vi "Formular Analyze.vi"(8 "error in (no error)":errorcluster caption="Error In", 10 "Formular":string="EL_A/(SY_Pieces*SY_Activation_Area)", 11 "Project":string) -> (0 "error out":errorcluster caption="Error Out", 1 "Value":string[](array[string]), 2 "Parameter":string[](array[string]), 3 "Result":string, 5 "Value":dbl)   [LabVIEW 2020]
uses:
  Global/Data Global/Data Global Mode.ctl
  375d7d93-2e26-4f59-bd85-31ccd4dbf3b0.vi
  <vilib>/regexp/Match Regular Expression.xnode
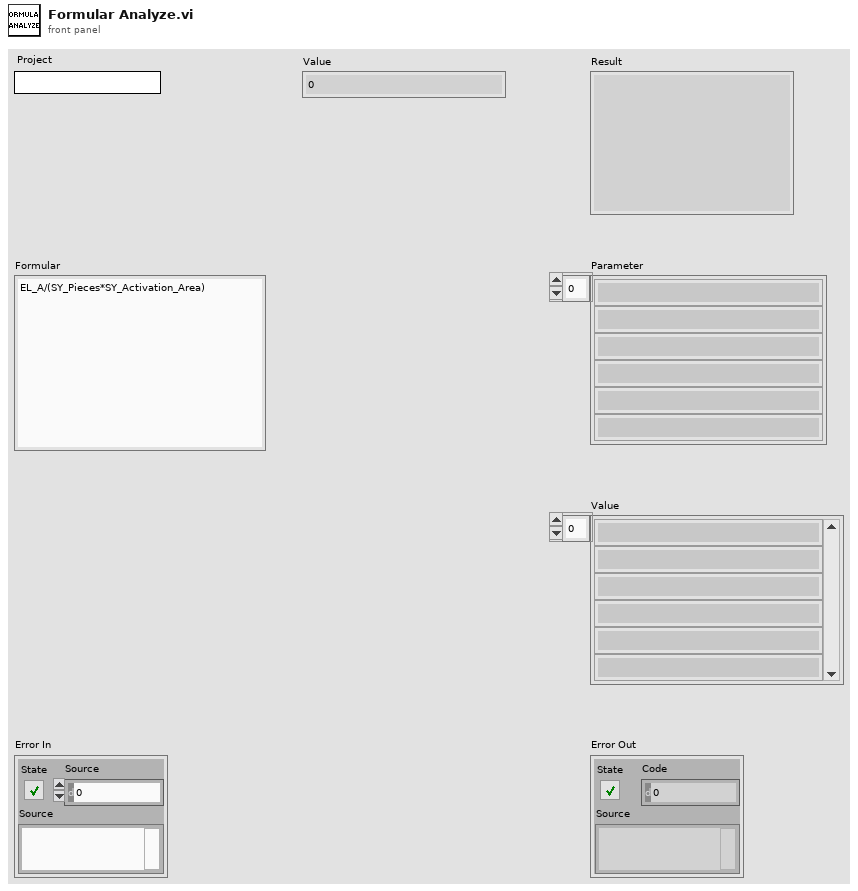
[diagram p1: front panel]
types:
  T1 = typedef "Data Global Mode.ctl" = enum16{"Init", "Read", "Write", "Write Data", "Load"}
  T2 = typedef "SDQ Data Type.ctl" = cluster{"CAN Length":string, "CAN Name":string, "CAN ID":string, "CAN Type":string, "Test Item":string, "Byte Order":string, "Instruction":string, "Control Type":string, "Group":string, "Offset":dbl, "Coefficient":dbl, "Write Enable":bool, "Lable Type":string, "Key?":string, "Set Value":string, "Upper":dbl, "Lower":dbl, "Unit":string, "Formula":string, "Test Item Type":string, "Length":i32, "Address":string, "Name":string, "Identifier":string, "Data Type":string, "Enumerate?":string, "Enumerate List":string, "Data":string, "Source":string}
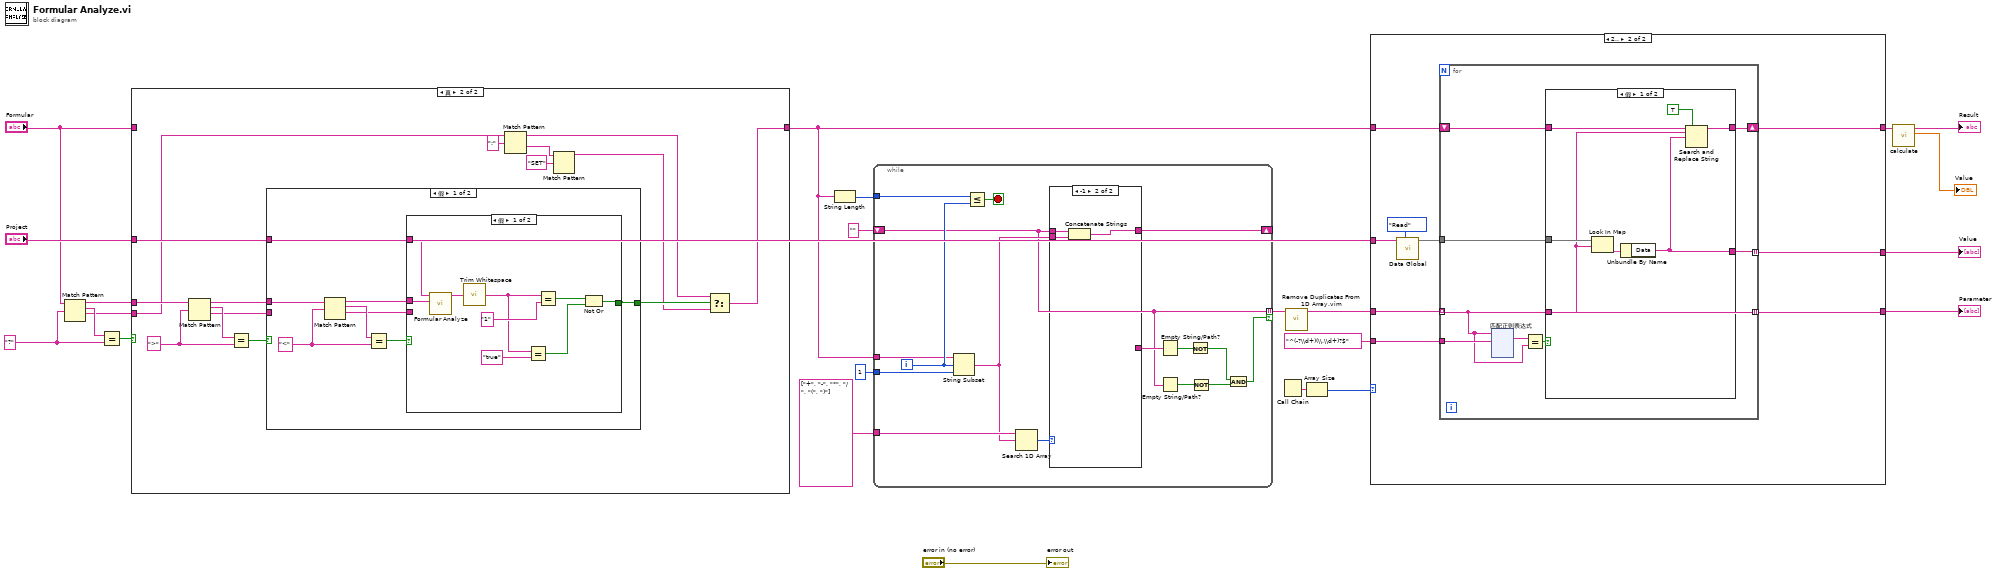
[diagram p0: block diagram]
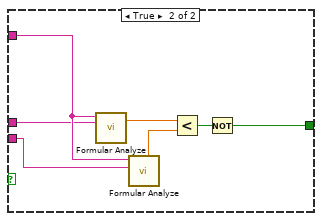
[diagram p3: hidden frame]
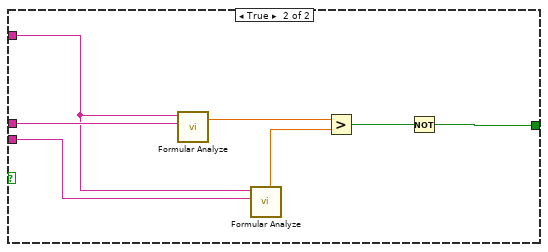
[diagram p4: hidden frame]
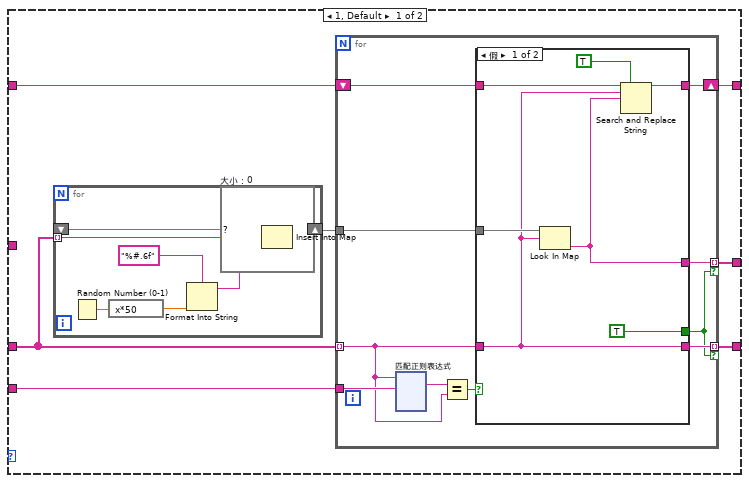
[diagram p5: hidden frame]
diagram:
  w10 = "?" ("正则表达式")
  n1 = Match Pattern(string="Formular", regular expression=w10) -> (before substring=w7:string, match substring=w11:string, after substring=w4:string)  [unwired: 1 in, 1 out]
  n2 = Equal?(x=w11, y=w10) -> (x = y?=w9:bool)
  n3 = case shown="真" w9 {
    tunnel: w7 -> [_ w39]
    tunnel: "Project" -> [_ w33]
    tunnel: w4 -> [_ w31]
    tunnel: "Formular" -> [w24 _]
    tunnel: [w24 w29] -> w2
    frame False {
    }
    frame True {
      w37 = ">" ("字符串")
      n4 = Match Pattern(string=w39, regular expression=w37) -> (before substring=w35:string, match substring=w38:string, after substring=w34:string)  [unwired: 1 in, 1 out]
      n5 = Equal?(x=w38, y=w37) -> (x = y?=w36:bool)
      n6 = case shown="假" w36 {
        tunnel: w35 -> [w47 w67]
        tunnel: w34 -> [_ w68]
        tunnel: w33 -> [w40 w66]
        tunnel: [w41 w64] -> w28
        frame False {
          w45 = "<" ("正则表达式")
          n7 = Match Pattern(string=w47, regular expression=w45) -> (before substring=w43:string, match substring=w46:string, after substring=w42:string)  [unwired: 1 in, 1 out]
          n8 = Equal?(x=w46, y=w45) -> (x = y?=w44:bool)
          n9 = case shown="假" w44 {
            tunnel: w43 -> [w49 w60]
            tunnel: w42 -> [_ w59]
            tunnel: [w52 w57] -> w41
            tunnel: w40 -> [w50 w61]
            frame False {
              n10 = call "Formular Analyze.vi"("Formular"=w49, "Project"=w50) -> ("Result"=w48:string)  [unwired: 5 in, 4 out]
              n11 = call <vilib>:"Trim Whitespace.vi"("string"=w48) -> ("trimmed string"=w51:string)  [unwired: 1 in]
              n12 = Equal?(x=w51, y="true") -> (x = y?=w53:bool)
              n13 = Equal?(x=w51, y="1") -> (x = y?=w54:bool)
              n14 = Not Or(1:w53, 2:w54) -> (0:w52:bool)
            }
            frame True {
              n15 = call "Formular Analyze.vi"("Formular"=w60, "Project"=w61) -> ("Value"=w63:dbl)  [unwired: 5 in, 4 out]
              n16 = call "Formular Analyze.vi"("Formular"=w59, "Project"=w61) -> ("Value"=w62:dbl)  [unwired: 5 in, 4 out]
              n17 = Less?(x=w63, y=w62) -> (x < y?=w58:bool)
              n18 = Not(x=w58) -> (.not. x?=w57:bool)
            }
          }
        }
        frame True {
          n19 = call "Formular Analyze.vi"("Formular"=w67, "Project"=w66) -> ("Value"=w70:dbl)  [unwired: 5 in, 4 out]
          n20 = call "Formular Analyze.vi"("Formular"=w68, "Project"=w66) -> ("Value"=w69:dbl)  [unwired: 5 in, 4 out]
          n21 = Greater?(x=w70, y=w69) -> (0:w65:bool)
          n22 = Not(x=w65) -> (.not. x?=w64:bool)
        }
      }
      n23 = Match Pattern(string=w31, regular expression=":" ("正则表达式")) -> (before substring=w30:string, after substring=w27:string)  [unwired: 1 in, 2 out]
      n24 = Match Pattern(string=w27, regular expression="SET" ("正则表达式")) -> (before substring=w25:string)  [unwired: 1 in, 3 out]
      n25 = Select(t=w30, s=w28, f=w25) -> (s? t:f=w29:string)
    }
  }
  n26 = String Length(string=w2) -> (length=w22:i32)
  n27 = while {
    tunnel: string[] ["+", "-", "*", "/", "(", ")"] -> [w82]
    tunnel: w22 -> [w86]
    tunnel: 1 ("长度（剩余）") -> [w83]
    shift-right: [w81] -> _
    shift-left: "" -> [w74]
    tunnel: [w74] -> w8 mode=indexing if=w72
    tunnel: w2 -> [w79]
    i -> [w84]
    stop <- w85 stop-if-true
    n28 = String Subset(string=w79, offset (0)=w84, length (rest)=w83) -> (substring=w77:string)
    n29 = Less Or Equal?(x=w86, y=w84) -> (x <= y?=w85:bool)
    n30 = Search 1D Array(1D array=w82, element=w77) -> (index of element=w78:i32)  [unwired: 1 in]
    n31 = case shown="-1" w78 {
      tunnel: w74 -> [_ w90]
      tunnel: w77 -> [w87 w89]
      tunnel: [_ w88] -> w81
      tunnel: [w87 _] -> w76
      frame 0, Default {
      }
      frame -1 {
        n32 = Concatenate Strings(w90, w89) -> (w88:string)
      }
    }
    n33 = Empty String/Path?(string/path=w76) -> (empty?=w80:bool)
    n34 = Empty String/Path?(string/path=w74) -> (empty?=w75:bool)
    n35 = Not(x=w80) -> (.not. x?=w71:bool)
    n36 = Not(x=w75) -> (.not. x?=w73:bool)
    n37 = And(x=w71, y=w73) -> (x .and. y?=w72:bool)
  }
  n38 = Call Chain() -> (call chain=w18:string[])
  n39 = call "Remove Duplicates From 1D Array.vim"("array"=w8) -> ("array with duplicates removed"=w15:string[])  [unwired: 10 in]
  n40 = Array Size(array=w18) -> (size(s)=w17:i32)
  n41 = case shown="2.." w17 {
    tunnel: w15 -> [w94 w245]
    tunnel: w2 -> [w96 w244]
    tunnel: [w95 w243] -> w16
    tunnel: [w91 w242] -> w12
    tunnel: [w93 w241] -> w13
    tunnel: "Project" -> [_ w240]
    tunnel: "^(-?\\d+)(\\.\\d+)?$" ("正则表达式") -> [w92 w239]
    frame 1, Default {
      w98 = map{string, string} {}  # 大小：0
      n42 = for {
        tunnel: w94 -> [w237] mode=indexing
        shift-right: [w235] -> w97
        shift-left: w98 -> [w238]
        n43 = Random Number (0-1)() -> (number: 0 to 1=w236:dbl)
        n44 = expression code="x*50"(w236) -> (w233:dbl)
        n45 = Format Into String(format string="%#.6f" ("格式字符串"), w233) -> (resulting string=w232:string)  [unwired: 2 in, 1 out]
        n46 = Insert Into Map(map in=w238, key=w237, value=w232) -> (map out=w235:map{string, string})  [unwired: 2 out]
      }
      n47 = for {
        tunnel: w97 -> [w108]
        tunnel: w94 -> [w101] mode=indexing
        shift-right: [w106] -> w95
        shift-left: w96 -> [w107]
        tunnel: [w105] -> w93 mode=indexing if=w99
        tunnel: w92 -> [w103]
        tunnel: [w100] -> w91 mode=indexing if=w99
        n48 = xnode "匹配正则表达式"("输入字符串"=w101, "正则表达式"=w103) -> ("所有匹配"=w104:string)  [unwired: 4 in, 4 out]
        n49 = Equal?(x=w104, y=w101) -> (x = y?=w102:bool)
        n50 = case shown="假" w102 {
          tunnel: w108 -> [w115 _]
          tunnel: w107 -> [w113 w117]
          tunnel: [w112 w117] -> w106
          tunnel: [w111 w116] -> w105
          tunnel: w101 -> [w109 w116]
          tunnel: [TRUE _] -> w99
          tunnel: [w109 _] -> w100
          frame False {
            n51 = Look In Map(map=w115, key=w109) -> (value=w111:string)  [unwired: 1 in, 1 out]
            n52 = Search and Replace String(replace all?=TRUE ("替换全部？(F)"), input string=w113, search string=w109, replace string=w111) -> (result string=w112:string)  [unwired: 4 in, 3 out]
          }
          frame True {
          }
        }
      }
    }
    frame 2.. {
      n53 = call "Data Global.vi"("Operate"=Data_Global_Mode."Read", "Name"=w240) -> ("Data Out"=w246:map{string, T2})  [unwired: 6 in, 3 out]
      n54 = for {
        tunnel: w246 -> [w255]
        tunnel: w245 -> [w249] mode=indexing
        shift-right: [w253] -> w243
        shift-left: w244 -> [w254]
        tunnel: [w249] -> w242 mode=indexing
        tunnel: [w252] -> w241 mode=indexing
        tunnel: w239 -> [w250]
        n55 = xnode "匹配正则表达式"("输入字符串"=w249, "正则表达式"=w250) -> ("所有匹配"=w251:string)  [unwired: 4 in, 4 out]
        n56 = Equal?(x=w251, y=w249) -> (x = y?=w248:bool)
        n57 = case shown="假" w248 {
          tunnel: w255 -> [w262 _]
          tunnel: w254 -> [w259 w264]
          tunnel: [w258 w264] -> w253
          tunnel: [w257 w263] -> w252
          tunnel: w249 -> [w256 w263]
          frame False {
            n58 = Look In Map(map=w262, key=w256) -> (value=w261:T2)  [unwired: 1 in, 1 out]
            n59 = Unbundle By Name(w261) -> ("Data"=w257:string)
            n60 = Search and Replace String(replace all?=TRUE ("替换全部？(F)"), input string=w259, search string=w256, replace string=w257) -> (result string=w258:string)  [unwired: 4 in, 3 out]
          }
          frame True {
          }
        }
      }
    }
  }
  "Value" <- w13
  "Parameter" <- w12
  n61 = call "calculate.vi"("Formular"=w16) -> ("Value"=→"Value":dbl, "Result"=→"Result":string)  [unwired: 9 in]
  "error out" <- "error in (no error)"
